vi "Helper - Overlay waypoints.vi"(9 "Shape to Overlay":bool[][](array[boolean])=[[TRUE, TRUE, TRUE, TRUE, TRUE, TRUE, TRUE, FALSE, FALSE, FALSE, TRUE, TRUE, TRUE, TRUE, TRUE, TRUE, TRUE, FALSE], [TRUE, TRUE, TRUE, TRUE, TRUE, TRUE, FALSE, FALSE, FALSE, FALSE, FALSE, TRUE, TRUE, TRUE, TRUE, TRUE, TRUE, FALSE], [TRUE, TRUE, TRUE, TRUE, TRUE, FALSE, FALSE, TRUE, TRUE, TRUE, FALSE, FALSE, TRUE, TRUE, TRUE, TRUE, TRUE, FALSE], [TRUE, TRUE, TRUE, TRUE, FALSE, FALSE, FALSE, TRUE, TRUE, TRUE, FALSE, FALSE, FALSE, TRUE, TRUE, TRUE, TRUE, FALSE], [TRUE, TRUE, TRUE, FALSE, FALSE, FALSE, FALSE, TRUE, TRUE, TRUE, FALSE, FALSE, FALSE, FALSE, TRUE, TRUE, TRUE, FALSE], [TRUE, TRUE, FALSE, FALSE, FALSE, FALSE, FALSE, TRUE, TRUE, TRUE, FALSE, FALSE, FALSE, FALSE, FALSE, TRUE, TRUE, FALSE], [TRUE, FALSE, FALSE, FALSE, FALSE, FALSE, FALSE, TRUE, TRUE, TRUE, FALSE, FALSE, FALSE, FALSE, FALSE, FALSE, TRUE, FALSE], [FALSE, FALSE, TRUE, TRUE, TRUE, TRUE, TRUE, TRUE, TRUE, TRUE, TRUE, TRUE, TRUE, TRUE, TRUE, FALSE, FALSE, FALSE], [FALSE, FALSE, TRUE, TRUE, TRUE, TRUE, TRUE, TRUE, TRUE, TRUE, TRUE, TRUE, TRUE, TRUE, TRUE, FALSE, FALSE, FALSE], [FALSE, FALSE, TRUE, TRUE, TRUE, TRUE, TRUE, TRUE, TRUE, TRUE, TRUE, TRUE, TRUE, TRUE, TRUE, FALSE, FALSE, FALSE], [TRUE, FALSE, FALSE, FALSE, FALSE, FALSE, FALSE, TRUE, TRUE, TRUE, FALSE, FALSE, FALSE, FALSE, FALSE, FALSE, TRUE, FALSE], [TRUE, TRUE, FALSE, FALSE, FALSE, FALSE, FALSE, TRUE, TRUE, TRUE, FALSE, FALSE, FALSE, FALSE, FALSE, TRUE, TRUE, FALSE], [TRUE, TRUE, TRUE, FALSE, FALSE, FALSE, FALSE, TRUE, TRUE, TRUE, FALSE, FALSE, FALSE, FALSE, TRUE, TRUE, TRUE, FALSE], [TRUE, TRUE, TRUE, TRUE, FALSE, FALSE, FALSE, TRUE, TRUE, TRUE, FALSE, FALSE, FALSE, TRUE, TRUE, TRUE, TRUE, FALSE], [TRUE, TRUE, TRUE, TRUE, TRUE, FALSE, FALSE, TRUE, TRUE, TRUE, FALSE, FALSE, TRUE, TRUE, TRUE, TRUE, TRUE, FALSE], [TRUE, TRUE, TRUE, TRUE, TRUE, TRUE, FALSE, FALSE, FALSE, FALSE, FALSE, TRUE, TRUE, TRUE, TRUE, TRUE, TRUE, FALSE], [TRUE, TRUE, TRUE, TRUE, TRUE, TRUE, TRUE, FALSE, FALSE, FALSE, TRUE, TRUE, TRUE, TRUE, TRUE, TRUE, TRUE, FALSE]], 10 "Color to Overlay":u32(colorbox)=16711680, 11 "Img Refnum in":T1) -> (3 "Img Refnum out":T1)   [LabVIEW 2011]
doc: "Given an image, reads the current list of waypoints off of the global variable and overlays their UTM-to-pixel conversions on the image.\n\nPurpose: Allows us to see our waypoints on an overview map or overhead camera image.\n\nAuthor: Jason Curtis"
uses:
  <vilib>/vision/Image Controls.llb/IMAQ Image.ctl
  2 Globals/2 Global.vi
panel:
  out "overlayed locations":cluster{"X":i32, "Y":i32}[](array[cluster])
  out "Bitmap to overlay":u32[][](array[colorbox])
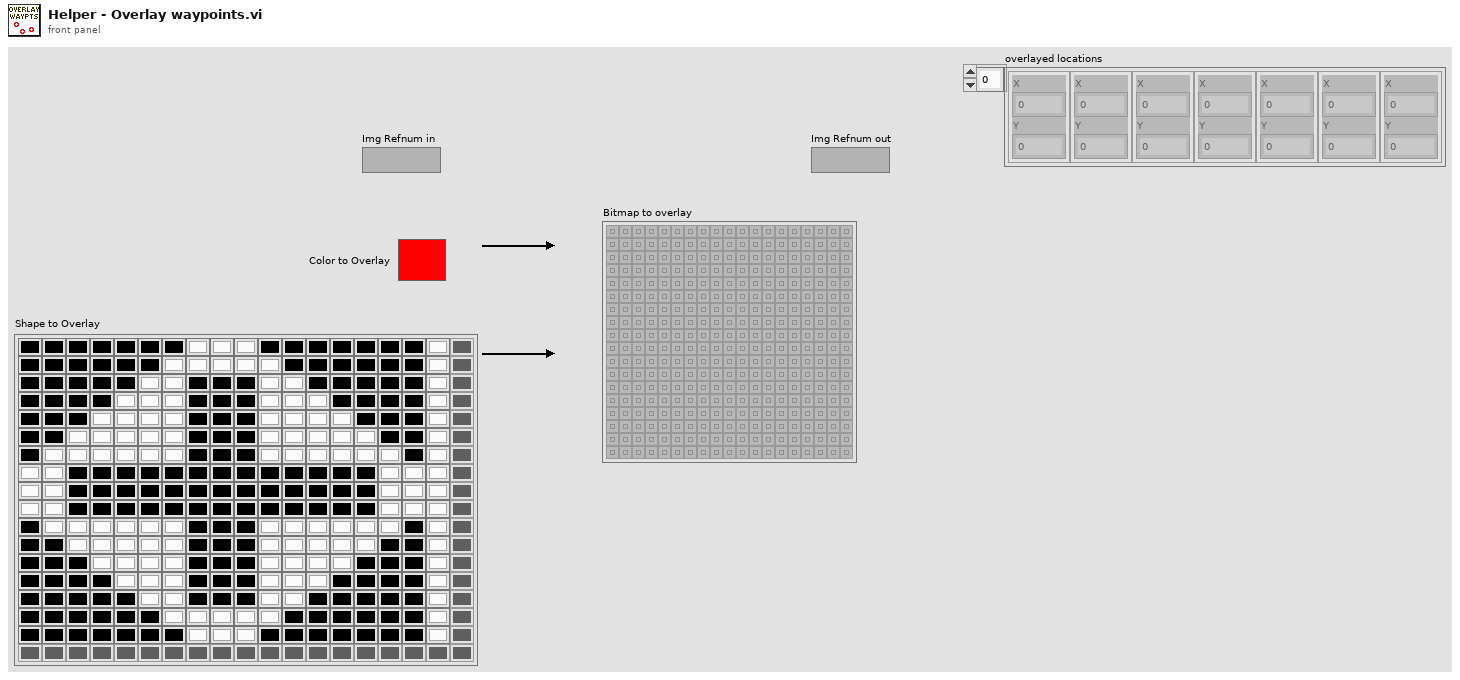
[diagram p1: front panel]
types:
  T1 = typedef "IMAQ Image.ctl" = refnum<image>
  T2 = typedef "ocuWaypoints.ctl" = cluster{"Waypoints Array":T3[], "Current Waypoint":dbl}
  T3 = typedef "ocuWaypoint.ctl" = cluster{"Point Type":T4, "Dist/Time":dbl, "UTM Location":T5}
  T4 = typedef "waypointTypes.ctl" = u16
  T5 = typedef "UTM Location.ctl" = cluster{"UTM Zone":dbl, "Hemisphere":enum16{"North", "South"}, "East":dbl, "North":dbl}
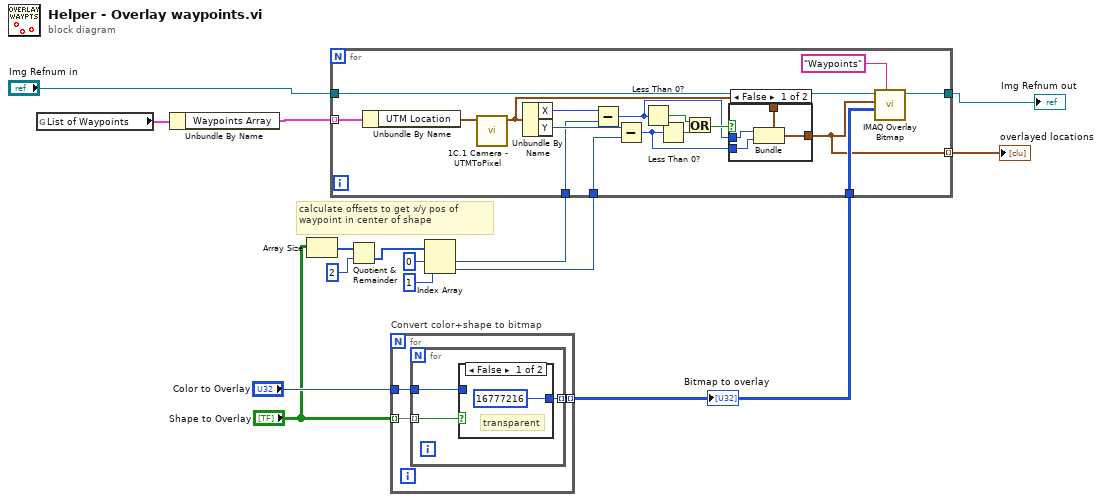
[diagram p0: block diagram]
diagram:
  # "calculate offsets to get x/y pos of waypoint in center of shape"
  n1 = global read "2 Global.vi" "List of Waypoints"() -> (w14:T2)
  n2 = Unbundle By Name(w14) -> ("Waypoints Array"=w13:T3[])
  n3 = Array Size(array="Shape to Overlay") -> (size(s)=w5:i32[])
  n4 = Quotient & Remainder(x=w5, y=2 ("index")) -> (floor(x/y)=w3:i32[])  [unwired: 1 out]
  n5 = for "Convert color+shape to bitmap" {
    tunnel: "Shape to Overlay" -> [w18] mode=indexing
    tunnel: [w17] -> w10 mode=indexing
    tunnel: "Color to Overlay" -> [w16]
    n6 = for {
      tunnel: w18 -> [w21] mode=indexing
      tunnel: [w20] -> w17 mode=indexing
      tunnel: w16 -> [w19]
      n7 = case shown="False" w21 {
        tunnel: [u32 16777216 ("element") w23] -> w20
        tunnel: w19 -> [_ w23]
        frame False {
          # "transparent"
        }
        frame True {
        }
      }
    }
  }
  "Bitmap to overlay" <- w10
  n8 = Index Array(array=w3, index #1=0 ("index"), index #2=1 ("index")) -> (element #1=w2:i32, element #2=w6:i32)
  n9 = for {
    tunnel: "Img Refnum in" -> [w37]
    tunnel: [w38] -> w12
    tunnel: w13 -> [w40] mode=indexing
    tunnel: w10 -> [w35]
    tunnel: w2 -> [w33]
    tunnel: w6 -> [w32]
    tunnel: [w25] -> w1 mode=indexing
    n10 = Unbundle By Name(w40) -> ("UTM Location"=w39:T5)
    n11 = call "1C.1 Camera - UTMToPixel.vi"("Robot UTM Location in"=w39) -> ("output pixels cluster"=w24:cluster{"X":i32, "Y":i32})  [unwired: 10 in]
    n12 = Unbundle By Name(w24) -> ("X"=w31:i32, "Y"=w34:i32)
    n13 = Subtract(x=w31, y=w33) -> (x-y=w27:i32)
    n14 = Subtract(x=w34, y=w32) -> (x-y=w26:i32)
    n15 = Less Than 0?(x=w27) -> (x < 0?=w30:bool)
    n16 = Less Than 0?(x=w26) -> (x < 0?=w29:bool)
    n17 = Or(x=w30, y=w29) -> (x .or. y?=w28:bool)
    n18 = case shown="False" w28 {
      tunnel: w24 -> [w44 w45]
      tunnel: w27 -> [w43 _]
      tunnel: w26 -> [w42 _]
      tunnel: [w41 w45] -> w25
      frame False {
        n19 = Bundle(cluster=w44, "X"=w43, "Y"=w42) -> (w41:cluster{"X":i32, "Y":i32})
      }
      frame True {
      }
    }
    n20 = call "IMAQ Overlay Bitmap"("Group"="Waypoints", "Bitmap"=w35, "Top Left Point"=w25, "Image"=w37) -> ("Image Out"=w38:T1)  [unwired: 6 in, 1 out]
  }
  "Img Refnum out" <- w12
  "overlayed locations" <- w1
